vi "IV and Differential Resistances.vi"(2 "Derivative Interval":i32=5 min=0, 3 "Electrical Measurement":T2) -> (0 "Differential Resistances":T1(array[cluster]), 1 "Current Voltage-Characteristics":cluster{"Voltage":dbl[], "Current":dbl[]}[](array[cluster]))   [LabVIEW 2014]
uses:
  <vilib>/Analysis/baseanly.llb/Mean (DBL).vi
  <vilib>/Analysis/NI_AALPro.lvlib
  <vilib>/Analysis/NI_AALBase.lvlib
panel:
  # "LICENSED MATERIALS – PROPERTY OF IBM\nCopyright IBM Corp. 2016,\nALL RIGHTS RESERVED"
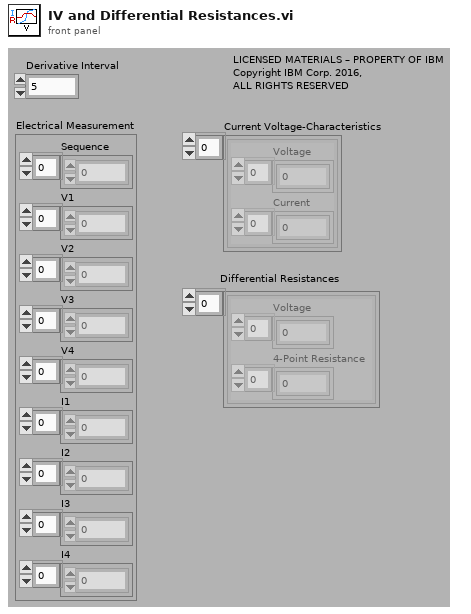
[diagram p1: front panel]
types:
  T1 = cluster{"Voltage":dbl[], "4-Point Resistance":dbl[]}[]
  T2 = cluster{"Sequence":dbl[], "V1":dbl[], "V2":dbl[], "V3":dbl[], "V4":dbl[], "I1":dbl[], "I2":dbl[], "I3":dbl[], "I4":dbl[]}
  T3 = cluster{"Voltage":dbl[], "4-Point Resistance":dbl[]}
  T4 = cluster{"Voltage":dbl[], "2-Point Resistance":dbl[]}
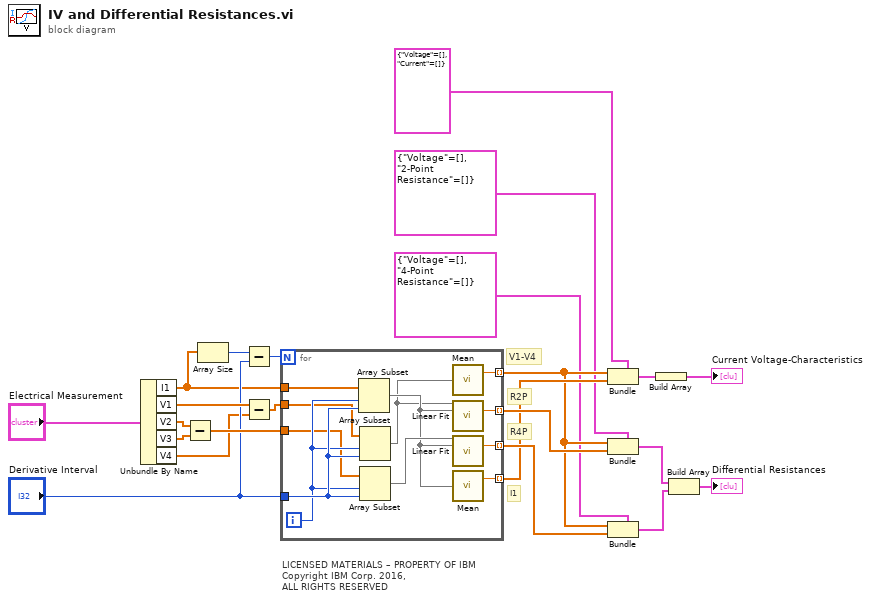
[diagram p0: block diagram]
diagram:
  # "LICENSED MATERIALS – PROPERTY OF IBM\nCopyright IBM Corp. 2016,\nALL RIGHTS RESERVED"
  # "R4P"
  # "R2P"
  # "I1"
  # "V1-V4"
  n1 = Unbundle By Name("Electrical Measurement") -> ("I1"=w16:dbl[], "V1"=w22:dbl[], "V2"=w21:dbl[], "V3"=w20:dbl[], "V4"=w2:dbl[])
  n2 = Subtract(x=w21, y=w20) -> (x-y=w19:dbl[])
  n3 = Array Size(array=w16) -> (size(s)=w18:i32)
  n4 = Subtract(x=w18, y="Derivative Interval") -> (x-y=w15:i32)
  n5 = Subtract(x=w22, y=w2) -> (x-y=w3:dbl[])
  n6 = for {
    N: w15 -> [_]
    tunnel: "Derivative Interval" -> [w34]
    tunnel: w16 -> [w35]
    tunnel: w3 -> [w32]
    tunnel: w19 -> [w31]
    tunnel: [w28] -> w14 mode=indexing
    tunnel: [w27] -> w13 mode=indexing
    tunnel: [w26] -> w12 mode=indexing
    tunnel: [w24] -> w11 mode=indexing
    i -> [w33]
    n7 = Array Subset(array=w35, index=w33, length=w34) -> (w29:dbl[])
    n8 = Array Subset(array=w32, index=w33, length=w34) -> (w25:dbl[])
    n9 = Array Subset(array=w31, index=w33, length=w34) -> (w30:dbl[])
    n10 = call-poly <vilib>:"Mean.vi"("X"=w25) -> ("mean"=w24:dbl)  [unwired: 1 out]
    n11 = call <vilib>:"Linear Fit.vi"("Y"=w25, "X"=w29) -> ("slope"=w28:dbl)  [unwired: 4 in, 9 out]
    n12 = call <vilib>:"Linear Fit.vi"("Y"=w30, "X"=w29) -> ("slope"=w27:dbl)  [unwired: 4 in, 9 out]
    n13 = call-poly <vilib>:"Mean.vi"("X"=w29) -> ("mean"=w26:dbl)  [unwired: 1 out]
  }
  n14 = Bundle(cluster=cluster{"Voltage":dbl[], "Current":dbl[]} {"Voltage"=[], "Current"=[]}, "Voltage"=w11, "Current"=w12) -> (w7:cluster{"Voltage":dbl[], "Current":dbl[]})
  n15 = Bundle(cluster=T4 {"Voltage"=[], "2-Point Resistance"=[]}, "Voltage"=w11, "2-Point Resistance"=w14) -> (w5:T4)
  n16 = Bundle(cluster=T3 {"Voltage"=[], "4-Point Resistance"=[]}, "Voltage"=w11, "4-Point Resistance"=w13) -> (w1:T3)
  n17 = Build Array(w7) -> (→"Current Voltage-Characteristics":cluster{"Voltage":dbl[], "Current":dbl[]}[])
  n18 = Build Array(w5, w1) -> (→"Differential Resistances":T1)
